vi "CC linearity test.vi"() -> ()   [LabVIEW 2013]
uses:
  Control 2.ctl
  Control 3.ctl
  Control 4.ctl
  Control 5.ctl
  Control 6.ctl
  Control 1.ctl
panel:
  in  "Cal. factor":dbl=3.023
  in  "Code":u16
  in  "Use code":bool
  out "Voltage (V)":dbl format="%.5f"
  out "Current (mA)":dbl format="%.5f"
  in  "Start sweep":bool
  out "XY Graph":cluster{i32[], dbl[]}(graph)
  out "ADC Current":dbl caption="mA" format="%.4f"
  out "ADC Voltage":dbl caption="V" format="%.4f"
  in  "DAC output (V)":dbl(slide) scale=0.0..4.8
  out "Configuration byte":u8 format="%02x"
  in  "ADC Bit Depth selection":enum32{"CH1", "CH2", "CH2 2", "CH2 3"}(radio)=enum."CH2 2"
  in  "ADC Channel selection":enum32{"CH1", "CH2"}(radio)
  in  "Bit 16":T1
  in  "Bit 15":T2
  in  "Bit 14":T3
  in  "Bit 13":T4
  in  "Bit 12":T5
  in  "Bit 11":bool
  in  "Bit 9 - Cell on (inv.)":bool
  in  "Bit 10":bool
  in  "Bit 8":bool
  in  "Bit 7":bool
  in  "Bit 6":bool
  in  "Bit 5":bool
  in  "Bit 4":bool
  in  "Bit 3":bool
  in  "Bit 1":bool
  in  "Bit 2":bool
  in  "Stop":bool
  out "Iteration":i32
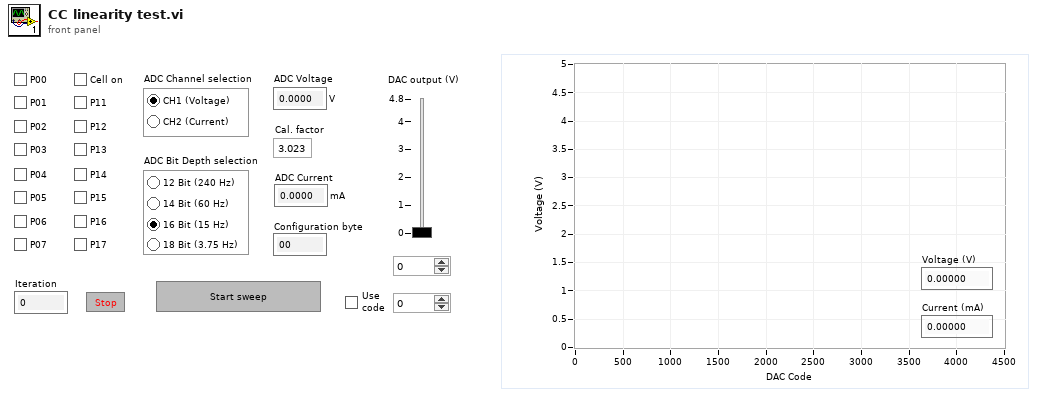
[diagram p1: front panel]
types:
  T1 = typedef "Control 6.ctl" = bool
  T2 = typedef "Control 5.ctl" = bool
  T3 = typedef "Control 4.ctl" = bool
  T4 = typedef "Control 3.ctl" = bool
  T5 = typedef "Control 2.ctl" = bool
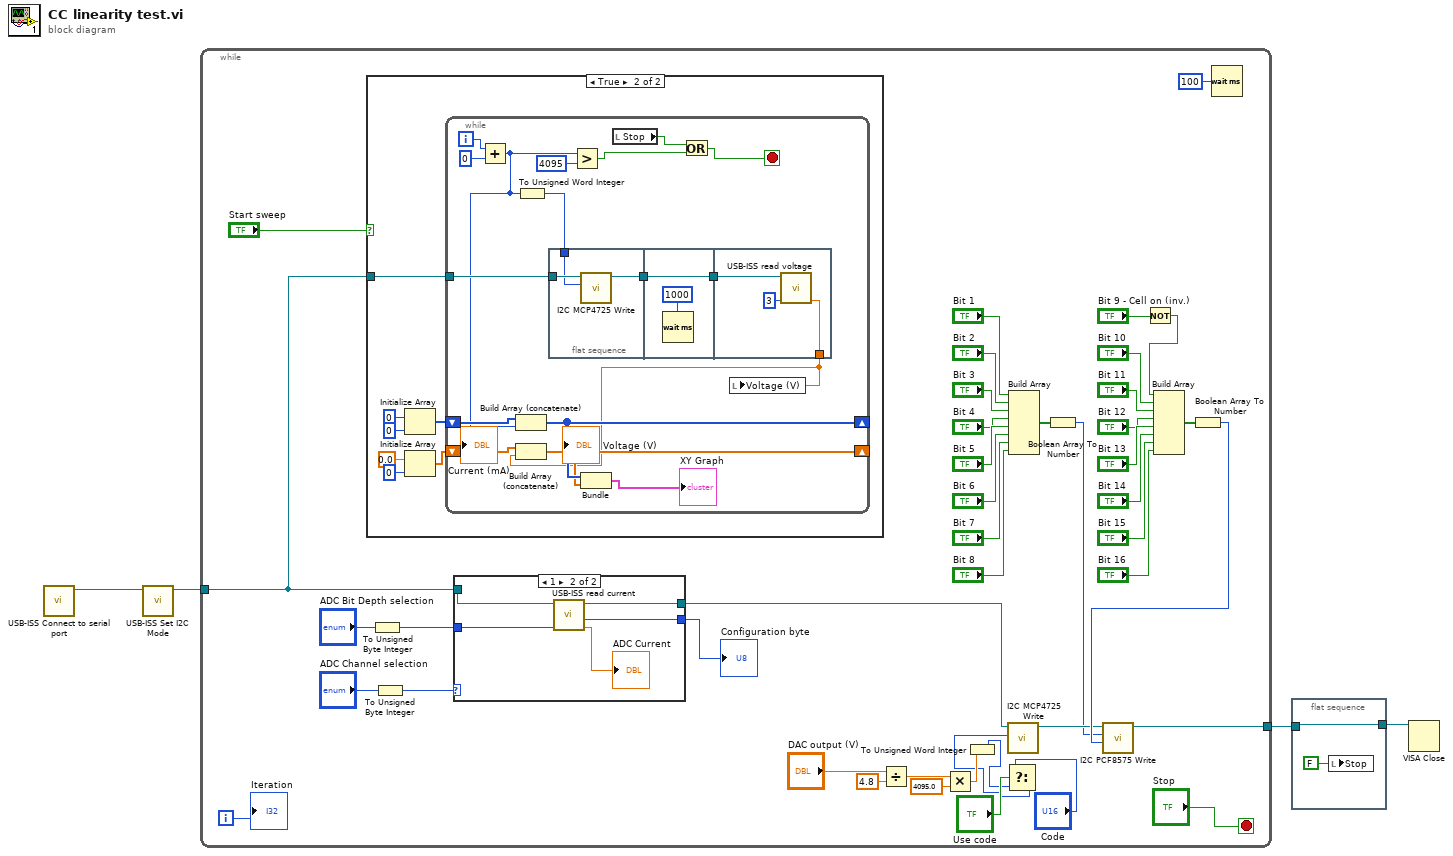
[diagram p0: block diagram]
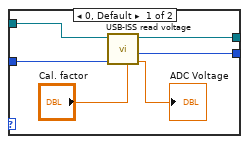
[diagram p3: hidden frame]
diagram:
  n1 = call "USB-ISS Connect to serial port.vi"() -> ("VISA Refnum out"=w3:refnum<visa-resource-name>)  [unwired: 10 in, 1 out]
  n2 = call "USB-ISS Set I2C Mode.vi"("VISA Refnum in"=w3) -> ("VISA Refnum out"=w4:refnum<visa-resource-name>)  [unwired: 9 in, 1 out]
  n3 = while {
    tunnel: [w46] -> w2
    tunnel: w4 -> [w6]
    i -> [w47]
    stop <- "Stop" stop-if-true
    n4 = case shown="True" "Start sweep" {
      tunnel: w6 -> [_ w48]
      frame False {
      }
      frame True {
        n5 = Initialize Array(0 ("element"), 0 ("dimension size")) -> (w54:i32[])
        n6 = Initialize Array(0.0 ("element"), 0 ("dimension size")) -> (w51:dbl[])
        n7 = while {
          tunnel: w48 -> [w71]
          shift-right: [w68] -> _
          shift-left: w54 -> [w70]
          shift-right: [w67] -> _
          shift-left: w51 -> [w69]
          i -> [w65]
          stop <- w56 stop-if-true
          n8 = Add(x=w65, y=0) -> (x+y=w62:i32)
          n9 = Build Array (concatenate)(w70, w62) -> (w68:i32[])
          n10 = Build Array (concatenate)(w69, w61) -> (w67:dbl[])
          n11 = To Unsigned Word Integer(number=w62) -> (unsigned 16bit integer=w58:u16)
          n12 = flat-sequence {
            tunnel: w71 -> [w74]
            tunnel: [w73] -> w60
            tunnel: w58 -> [w72]
            tunnel: w60 -> [w76]
            tunnel: [w76] -> w59
            tunnel: [w79] -> w61
            tunnel: w59 -> [w77]
            frame #0 {
              n13 = call "I2C MCP4725 Write.vi"("DAC code"=w72, "VISA Refnum in"=w74) -> ("VISA Refnum out"=w73:refnum<visa-resource-name>)  [unwired: 6 in, 1 out]
            }
            frame #1 {
              n14 = Wait (ms)(milliseconds to wait=u32 1000) -> ()  [unwired: 1 out]
            }
            frame #2 {
              n15 = call "USB-ISS read voltage.vi"("Bit depth"=u8 3, "VISA Refnum in"=w77) -> ("Voltage in V"=w79:dbl)  [unwired: 7 in, 2 out]
            }
          }
          n16 = Greater?(x=w62, y=4095) -> (0:w57:bool)
          n17 = Bundle(w68, w67) -> (→"XY Graph":cluster{i32[], dbl[]})  [unwired: 1 in]
          n18 = local read "Stop"() -> (w55:bool)
          n19 = Or(x=w55, y=w57) -> (x .or. y?=w56:bool)
          n20 = local write "Voltage (V)"(w61) -> ()
        }
      }
    }
    n21 = To Unsigned Byte Integer(number="ADC Bit Depth selection") -> (unsigned 8bit integer=w9:u8)
    n22 = To Unsigned Byte Integer(number="ADC Channel selection") -> (unsigned 8bit integer=w8:u8)
    n23 = case shown="1" w8 {
      tunnel: [w83 w90] -> w10
      tunnel: w9 -> [w82 w87]
      tunnel: w6 -> [w81 w88]
      tunnel: [w80 w89] -> w7
      frame 0, Default {
        n24 = call "USB-ISS read voltage.vi"("Calibration factor"="Cal. factor", "Bit depth"=w82, "VISA Refnum in"=w81) -> ("Voltage in V"=→"ADC Voltage":dbl, "Configuration byte"=w83:u8, "VISA Refnum out"=w80:refnum<visa-resource-name>)  [unwired: 6 in]
      }
      frame 1 {
        n25 = call "USB-ISS read current.vi"("Bit depth"=w87, "VISA Refnum in"=w88) -> ("Current in mA"=→"ADC Current":dbl, "Configuration byte"=w90:u8, "VISA Refnum out"=w89:refnum<visa-resource-name>)  [unwired: 7 in]
      }
    }
    "Configuration byte" <- w10
    n26 = Divide(x="DAC output (V)", y=4.8) -> (x/y=w19:dbl)
    n27 = Multiply(x=w19, y=4095.0) -> (x*y=w16:dbl)
    n28 = To Unsigned Word Integer(number=w16) -> (unsigned 16bit integer=w12:u16)
    n29 = Select(t="Code", s="Use code", f=w12) -> (s? t:f=w11:u16)
    n30 = call "I2C MCP4725 Write.vi"("DAC code"=w11, "VISA Refnum in"=w7) -> ("VISA Refnum out"=w22:refnum<visa-resource-name>)  [unwired: 6 in, 1 out]
    n31 = Build Array("Bit 1", "Bit 2", "Bit 3", "Bit 4", "Bit 5", "Bit 6", "Bit 7", "Bit 8") -> (w37:bool[])
    n32 = Boolean Array To Number(Boolean array=w37) -> (number=w17:u8)
    n33 = Not(x="Bit 9 - Cell on (inv.)") -> (.not. x?=w26:bool)
    n34 = Build Array(w26, "Bit 10", "Bit 11", "Bit 12", "Bit 13", "Bit 14", "Bit 15", "Bit 16") -> (w45:T1[])
    n35 = Boolean Array To Number(Boolean array=w45) -> (number=w28:u8)
    n36 = call "I2C PCF8575 Write.vi"("Byte 2"=w28, "Byte 1"=w17, "VISA Refnum in"=w22) -> ("VISA Refnum out"=w46:refnum<visa-resource-name>)  [unwired: 7 in, 1 out]
    n37 = Wait (ms)(milliseconds to wait=u32 100) -> ()  [unwired: 1 out]
    "Iteration" <- w47
  }
  n38 = flat-sequence {
    tunnel: w2 -> [w92]
    tunnel: [w92] -> w1
    frame #0 {
      n39 = local write "Stop"(FALSE ("Stop")) -> ()
    }
  }
  n40 = VISA Close(VISA resource name=w1) -> ()  [unwired: 1 in, 1 out]
